vi "AI_Channels.vi"(11 "DAQmx Device Name":tag) -> (3 "Array":tag[](array[tag]), 5 "# AI":dbl)   [LabVIEW 2011]
uses:
  C:/Program Files/National Instruments/LabVIEW 2011/resource/objmgr/daqmx.rc
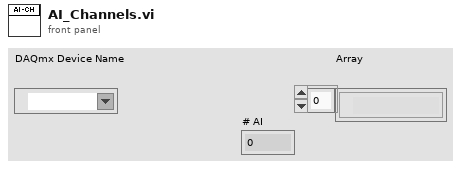
[diagram p1: front panel]
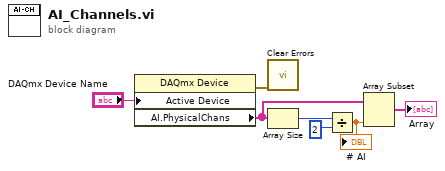
[diagram p0: block diagram]
diagram:
  n1 = property class="DAQmx Device"("Active Device"="DAQmx Device Name") -> (error out=w1:errorcluster, "AI.PhysicalChans"=w6:tag[])  [unwired: 2 in, 1 out]
  n2 = call "Clear Errors.vi"("error in (no error)"=w1) -> ()  [unwired: 6 in, 1 out]
  n3 = Array Size(array=w6) -> (size(s)=w2:i32)
  n4 = Divide(x=w2, y=2) -> (x/y=w4:dbl)
  "# AI" <- w4
  n5 = Array Subset(array=w6, length=w4) -> (→"Array":tag[])  [unwired: 1 in]
